vi "clear Multiple listbox.vi"(8 "Error In":errorcluster, 11 "Mutiple listbox reference in":refnum<vi>) -> (0 "Error Out":errorcluster, 3 "Mutiple listbox reference out":refnum<vi>)   [LabVIEW 2020]
doc: "Clean the mutiple listbox context"
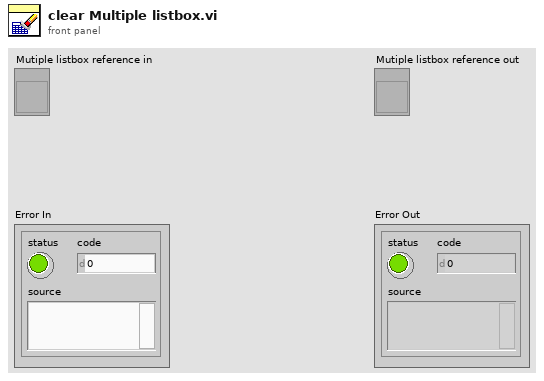
[diagram p1: front panel]
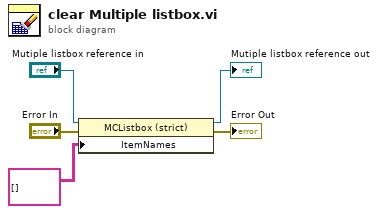
[diagram p0: block diagram]
diagram:
  n1 = property class="MCListbox (strict)"(reference="Mutiple listbox reference in", error in="Error In", "ItemNames"=string[][] [] ("Item Names")) -> (reference out=→"Mutiple listbox reference out":refnum<vi>, error out=→"Error Out":errorcluster)
